vi "Get Names.vi"(8 "error in (no error)":errorcluster, 11 "Blue Plugin in":refnum<class "Blue Plugin.lvclass">) -> (0 "error out":errorcluster, 2 "Name":string, 3 "Blue Plugin out":refnum<class "Blue Plugin.lvclass">)   [LabVIEW 2020, in "Blue Plugin.lvclass"]
uses:
  Blue Plugin.lvclass
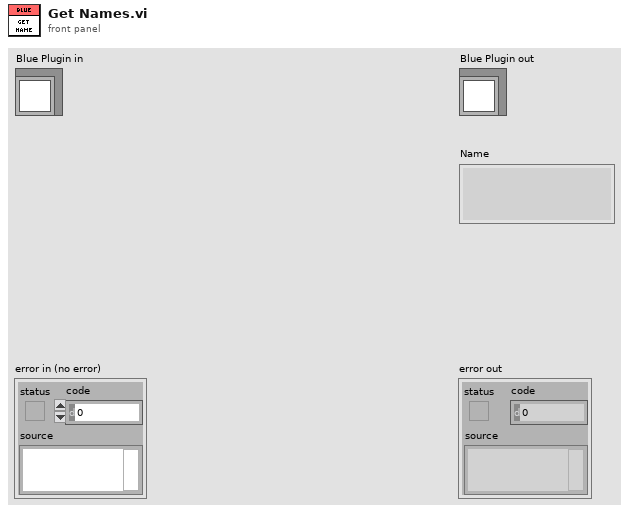
[diagram p1: front panel]
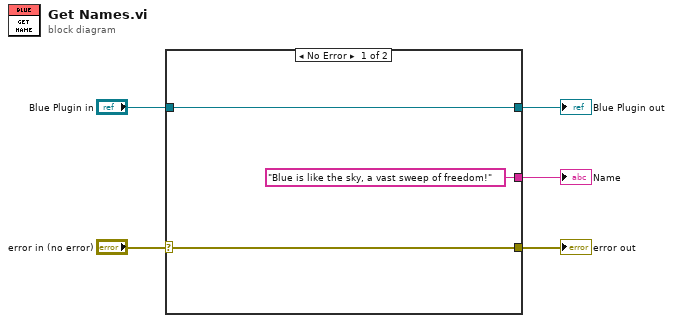
[diagram p0: block diagram]
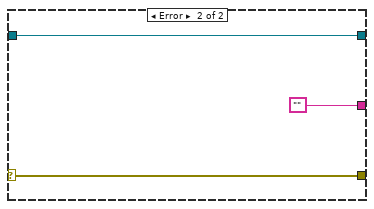
[diagram p2: hidden frame]
diagram:
  n1 = case shown="No Error" "error in (no error)" {
    selector: "error in (no error)" -> [w8 w11]
    tunnel: [w8 w11] -> w4
    tunnel: "Blue Plugin in" -> [w6 w10]
    tunnel: [w6 w10] -> w2
    tunnel: ["Blue is like the sky, a vast sweep of freedom!" ""] -> w1
    frame No Error {
    }
    frame Error {
    }
  }
  "error out" <- w4
  "Blue Plugin out" <- w2
  "Name" <- w1
